vi "Erase.vi"(8 "error in (no error)":errorcluster, 11 "DoubleLinkedList in":refnum<class "DoublyLinkedList.lvclass">) -> (0 "error out":errorcluster, 3 "DoubleLinkedList out":refnum<class "DoublyLinkedList.lvclass">)   [LabVIEW 2021, in "DoublyLinkedList.lvclass"]
uses:
  DoublyLinkedList.lvclass
  DoublyLinkedList.lvclass/DoublyLinkedList.ctl
  IDoublyNode/IDoublyNode.lvclass
  DoublyNode/DoublyNode.lvclass
panel:
  out "list node":refnum<class "DoublyNode.lvclass">
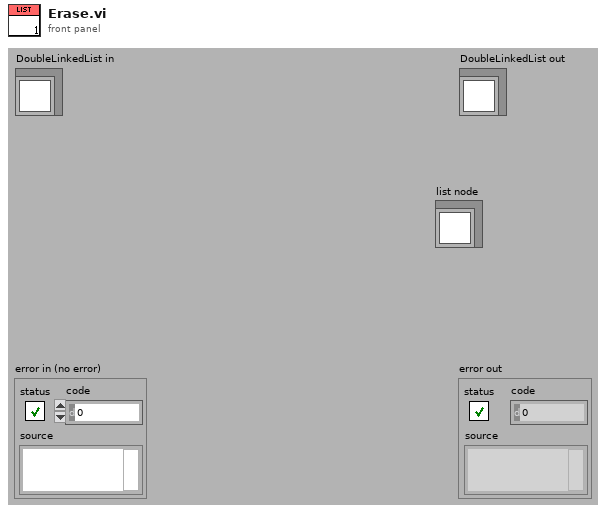
[diagram p1: front panel]
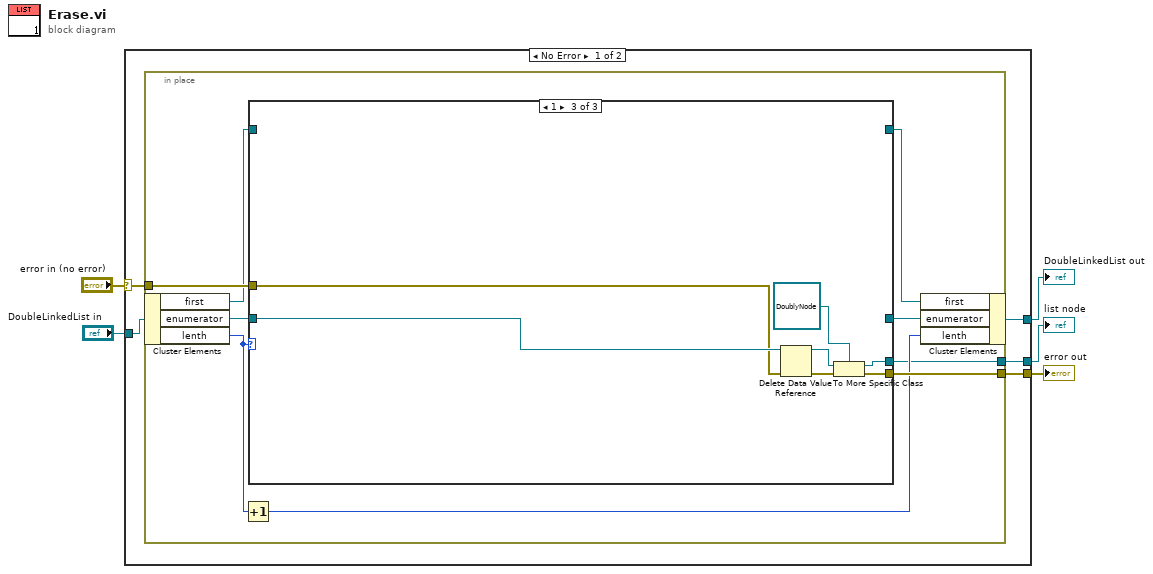
[diagram p0: block diagram]
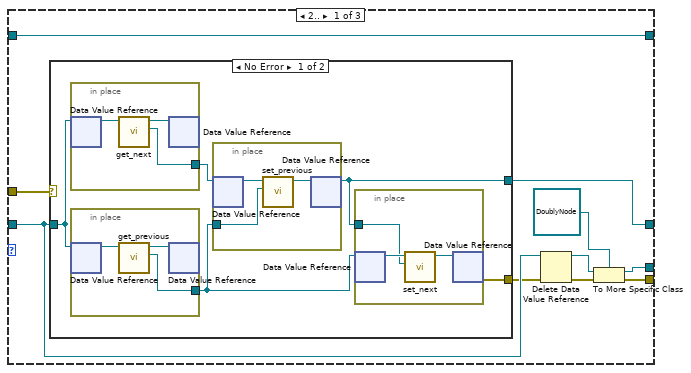
[diagram p2: hidden frame]
diagram:
  n1 = case shown="No Error" "error in (no error)" {
    selector: "error in (no error)" -> [w8 w60]
    tunnel: [w7 w60] -> w1
    tunnel: [w9 w59] -> w2
    tunnel: "DoubleLinkedList in" -> [w10 w59]
    tunnel: [w6 _] -> w4
    frame No Error {
      n2 = in-place {
        in-place-border: w8 -> [w17]
        in-place-border: [w16] -> w7
        in-place-border: [w11] -> w6
        n3 = in-place-cluster #1(w10) -> ("first"=w14:refnum<data-value>, "enumerator"=w19:refnum<data-value>, "lenth"=w12:u32)
        n4 = Increment(x=w12) -> (x+1=w13:u32)
        n5 = case shown="1" w12 {
          tunnel: w19 -> [w27 w51 w55]
          tunnel: [w28 w51 _] -> w18
          tunnel: w17 -> [w21 w50 w54]
          tunnel: [w20 w50 w53] -> w16
          tunnel: [w29 w49 _] -> w15
          tunnel: w14 -> [w29 w49 _]
          tunnel: [w23 _ w52] -> w11
          frame 2.. {
            n6 = case shown="No Error" w21 {
              selector: w21 -> [_ w48]
              tunnel: [w32 w47] -> w28
              tunnel: w27 -> [w31 w47]
              tunnel: [w30 w48] -> w26
              frame No Error {
                n7 = in-place {
                  in-place-border: [w45] -> w34
                  n8 = in-place-dvr #2(w31) -> (w46:refnum<class "IDoublyNode.lvclass">)  [unwired: 1 out]
                  n9 = call-dynamic "get_next.vi"("NodeType in"=w46) -> ("next"=w45:refnum<data-value>, "NodeType out"=w44:refnum<class "IDoublyNode.lvclass">)  [unwired: 8 in, 1 out]
                  n10 = in-place-dvr #2(w44) -> ()  [unwired: 2 out]
                }
                n11 = in-place {
                  in-place-border: [w42] -> w33
                  n12 = in-place-dvr #3(w31) -> (w43:refnum<class "IDoublyNode.lvclass">)  [unwired: 1 out]
                  n13 = call-dynamic "get_previous.vi"("NodeType in"=w43) -> ("previous"=w42:refnum<data-value>, "NodeType out"=w41:refnum<class "IDoublyNode.lvclass">)  [unwired: 8 in, 1 out]
                  n14 = in-place-dvr #3(w41) -> ()  [unwired: 2 out]
                }
                n15 = in-place {
                  in-place-border: w33 -> [w35]
                  n16 = in-place-dvr #4(w34) -> (w37:refnum<class "IDoublyNode.lvclass">)  [unwired: 1 out]
                  n17 = call-dynamic "set_previous.vi"("previous"=w35, "NodeType in"=w37) -> ("NodeType out"=w36:refnum<class "IDoublyNode.lvclass">)  [unwired: 8 in, 1 out]
                  n18 = in-place-dvr #4(w36) -> (w32:refnum<data-value>)  [unwired: 1 out]
                }
                n19 = in-place {
                  in-place-border: w32 -> [w38]
                  n20 = in-place-dvr #5(w33) -> (w40:refnum<class "IDoublyNode.lvclass">)  [unwired: 1 out]
                  n21 = call-dynamic "set_next.vi"("next"=w38, "NodeType in"=w40) -> ("NodeType out"=w39:refnum<class "IDoublyNode.lvclass">)  [unwired: 8 in, 1 out]
                  n22 = in-place-dvr #5(w39) -> (w30:errorcluster)  [unwired: 1 out]
                }
              }
              frame Error {
              }
            }
            n23 = Delete Data Value Reference(data value reference=w27, error in=w26) -> (data value=w24:refnum<class "IDoublyNode.lvclass">, error out=w22:errorcluster)
            n24 = To More Specific Class(target class=refnum<class "DoublyNode.lvclass"> refnum ("list node"), reference=w24, error in=w22) -> (specific class reference=w23:refnum<class "DoublyNode.lvclass">, error out=w20:errorcluster)
          }
          frame 0, Default {
          }
          frame 1 {
            n25 = Delete Data Value Reference(data value reference=w55, error in=w54) -> (data value=w57:refnum<class "IDoublyNode.lvclass">, error out=w56:errorcluster)
            n26 = To More Specific Class(target class=refnum<class "DoublyNode.lvclass"> refnum ("list node"), reference=w57, error in=w56) -> (specific class reference=w52:refnum<class "DoublyNode.lvclass">, error out=w53:errorcluster)
          }
        }
        n27 = in-place-cluster #1("first"=w15, "enumerator"=w18, "lenth"=w13) -> (w9:refnum<class "DoublyLinkedList.lvclass">)
      }
    }
    frame Error {
    }
  }
  "error out" <- w1
  "DoubleLinkedList out" <- w2
  "list node" <- w4
